vi "EFDUV Example Set Ultimus V Dispense Parameters.vi"(0 "VISA resource name":refnum<visa-resource-name>="COM1", 1 "Dispense Time":i32 format="%04.0f", 2 "Pressure Setting":i64 min=0 max=1000 step=1 format="%04.0f", 3 "Vacuum Setting":i64 min=0 max=1000 step=1 format="%04.0f", 4 "Vacuum Units":u16(ring)=1 items=["KPA", "inH2O", "inHg", "mmHg", "TORR"], 5 "Pressure Units":u16(ring) items=["PSI", "BAR", "KPA"], 6 "Auto Increment":u16(ring)=1 items=["Auto Increment OFF", "Timer Mode", "Counter Mode", "Auto Sequence Mode"], 7 "Set Start Address":i32 caption="Start" min=0 max=399 step=1 format="%03.0f", 8 "Dispense Mode":u16(ring) items=["Steady Mode", "Timed Mode"], 9 "Set End Address":i32=10 caption="Start" format="%03.0f", 10 "Serial Configuration":T1={"Baud Rate "=115200, "Parity "=0, "Data Bits "=8, "Stop Bits"=10} {"Stop Bits" items=["1.0"=10, "1.5"=15, "2.0"=20]; "Data Bits" items=["7"=7, "8"=8]; "Parity" items=["None", "Odd", "Even"]; "Baud Rate" items=["9600"=9600, "19200"=19200, "38400"=38400, "115200"=115200]}, 11 "Trigger Value (dddd)":i32=10 caption="Start" format="%03.0f") -> ()   [LabVIEW 2016]
doc: "Illustrates the ability to Set various parameters on the Ultimus V unit. Such as, Dispense mode, memory cell location, Time, Pressure, Vacuum, Auto Increment Mode etc."
uses:
  EFD Ultimus V.lvlib
panel:
  in  "Tab Control 2":enum32{"Set Parameters on the Ultimus V Unit"}(tab)
  in  "Memory Location":i32 min=0 max=399 step=1 format="%03.0f"
  # "3.Click the Run Button to update the Parameters on the\nUltimus V Unit."
  # "2.Select the Configuration Settings."
  # "1.Select the Serial Comm \nPort Associated with the \nUltimus V unit"
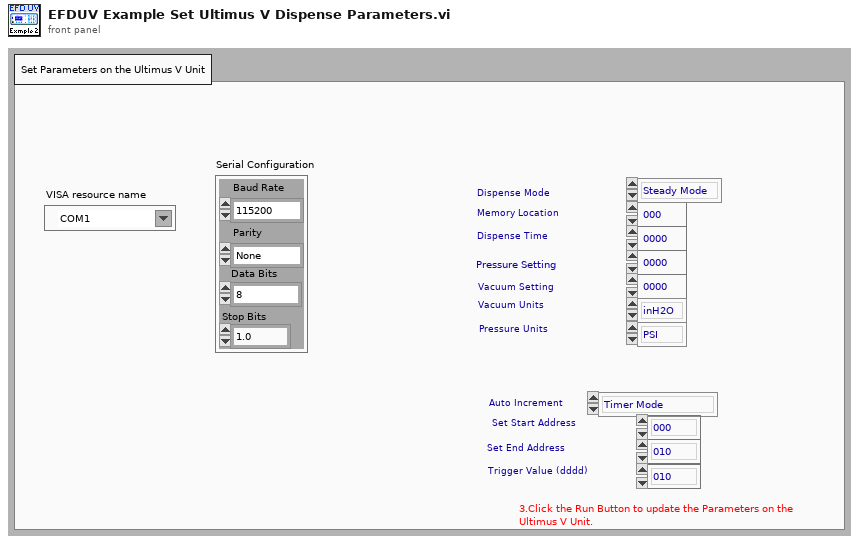
[diagram p1: front panel]
types:
  T1 = cluster{"Baud Rate ":u32, "Parity ":u16, "Data Bits ":u16, "Stop Bits":u16}
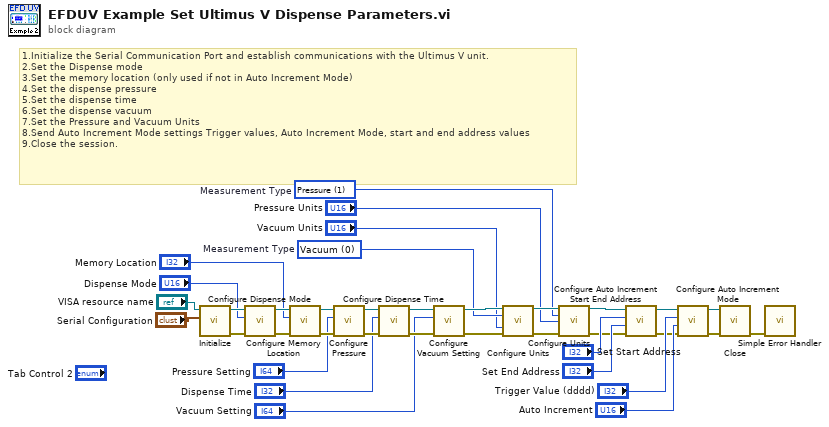
[diagram p0: block diagram]
diagram:
  w19 = u16 1 items=["Vacuum ", "Pressure"]  # Measurement Type
  w20 = u16 0 items=["Vacuum ", "Pressure"]  # Measurement Type
  # "1.Initialize the Serial Communication Port and establish communications with the Ultimus V unit.\n2.Set the Dispense mode \n3.Set the memory location (only used if not in Auto Increment Mode)\n4.Set the dispense pressure\n5.Set the dispense time\n6.Set the dispense vacuum\n7.Set the Pressure and Vacuum Units\n8.Send Auto Increment Mode settings Trigger values, Auto Increment Mode, start and end address values\n9.Close the session."
  n1 = call "Initialize.vi"("Serial Configuration"="Serial Configuration", "VISA resource name"="VISA resource name") -> ("error out"=w24:errorcluster, "VISA resource name out"=w23:refnum<visa-resource-name>)  [unwired: 8 in]
  n2 = call "Configure Dispense Mode.vi"("error in (no error)"=w24, "Dispense Mode (0: Steady)"="Dispense Mode", "VISA resource name"=w23) -> ("error out"=w34:errorcluster, "VISA resource name out"=w30:refnum<visa-resource-name>)  [unwired: 7 in]
  n3 = call "Configure Memory Location.vi"("error in (no error)"=w34, "Memory Location (000)"="Memory Location", "VISA resource name"=w30) -> ("error out"=w33:errorcluster, "VISA resource name out"=w29:refnum<visa-resource-name>)  [unwired: 7 in]
  n4 = call "Configure Pressure.vi"("error in (no error)"=w33, "Pressure Setting (0000)"="Pressure Setting", "VISA resource name"=w29) -> ("error out"=w32:errorcluster, "VISA resource name out"=w28:refnum<visa-resource-name>)  [unwired: 7 in]
  n5 = call "Configure Dispense Time.vi"("error in (no error)"=w32, "Dispense Time (0000)"="Dispense Time", "VISA resource name"=w28) -> ("error out"=w31:errorcluster, "VISA resource name out"=w27:refnum<visa-resource-name>)  [unwired: 7 in]
  n6 = call "Configure Vacuum Setting.vi"("error in (no error)"=w31, "Vacuum Setting (0000)"="Vacuum Setting", "VISA resource name"=w27) -> ("error out"=w26:errorcluster, "VISA resource name out"=w25:refnum<visa-resource-name>)  [unwired: 7 in]
  n7 = call "Configure Units.vi"("VISA resource name"=w25, "Measurement Type (0: Vacuum)"=w20, "Vacuum Units (1: inH20)"="Vacuum Units", "error in (no error)"=w26) -> ("VISA resource name out"=w22:refnum<visa-resource-name>, "error out"=w21:errorcluster)  [unwired: 10 in]
  n8 = call "Configure Units.vi"("VISA resource name"=w22, "Measurement Type (0: Vacuum)"=w19, "Pressure Units (0: PSI)"="Pressure Units", "error in (no error)"=w21) -> ("VISA resource name out"=w11:refnum<visa-resource-name>, "error out"=w12:errorcluster)  [unwired: 10 in]
  n9 = call "Configure Auto Increment Start End Address.vi"("error in (no error)"=w12, "End Address (000)"="Set End Address", "Start Address (000)"="Set Start Address", "VISA resource name"=w11) -> ("error out"=w9:errorcluster, "VISA resource name out"=w10:refnum<visa-resource-name>)  [unwired: 6 in]
  n10 = call "Configure Auto Increment Mode.vi"("error in (no error)"=w9, "Auto Increment (1:Timer)"="Auto Increment", "Trigger Value (0000)"="Trigger Value (dddd)", "VISA resource name"=w10) -> ("error out"=w7:errorcluster, "VISA resource name out"=w8:refnum<visa-resource-name>)  [unwired: 6 in]
  n11 = call "Close.vi"("error in (no error)"=w7, "VISA resource name"=w8) -> ("error out"=w6:errorcluster)  [unwired: 9 in]
  n12 = call <vilib>:"Simple Error Handler.vi"("error in (no error)"=w6) -> ()  [unwired: 4 in, 5 out]
